vi "Teardown.vi"(11 "Base Event in":refnum<class "Base Event.lvclass">) -> (3 "Base Event out":refnum<class "Base Event.lvclass">)   [LabVIEW 2021, in "jettl.lvlib" / "Base Event.lvlib" / "Base Event.lvclass"]
uses:
  Base Event.lvclass
  State/Teardown State/Teardown State.lvclass
  C:/git/jettl/src/jettl/Base Event/State/State/State.lvclass
  Base Event.lvclass/Base Event.ctl
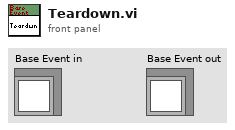
[diagram p1: front panel]
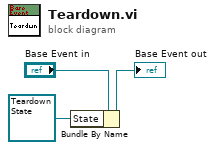
[diagram p0: block diagram]
diagram:
  n1 = Bundle By Name(cluster="Base Event in", "State"=refnum<class "Teardown State.lvclass"> refnum ("jettl.lvlib:Teardown Event State.lvclass")) -> (→"Base Event out":refnum<class "Base Event.lvclass">)
